vi "DAQ DO.vi"(8 "error in":errorcluster, 10 "on/off":bool, 11 "Alias":string="DO0") -> (0 "error out":errorcluster={"status"=TRUE, "code"=-200099, "source"="DAQmx Create Channel (DO-Digital Output).vi:6970001<append>\n<B>Task Name: </B>_unnamedTask<22>"})   [LabVIEW 2021]
uses:
  Controls/DAQ_Data.ctl
  <vilib>/DAQmx/write.llb/DAQmx Write (Digital Bool 1Line 1Point).vi
  <vilib>/DAQmx/create/channels.llb/DAQmx Create Channel (DO-Digital Output).vi
  <vilib>/DAQmx/miscellaneous.llb/DAQmx Fill In Error Info.vi
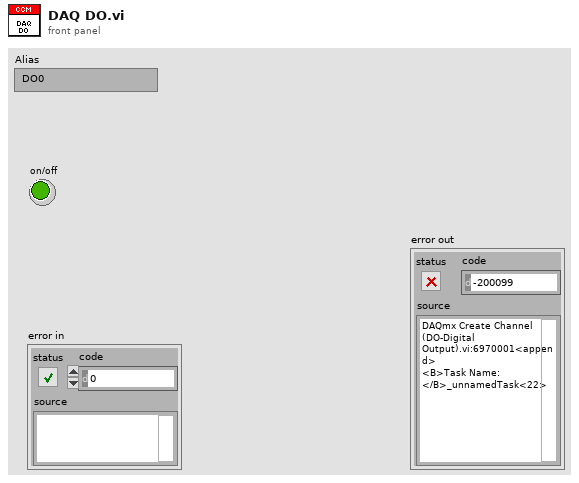
[diagram p1: front panel]
types:
  T1 = typedef "DAQ_Data.ctl" = cluster{"Alias":string, "DAQ Ch":string}
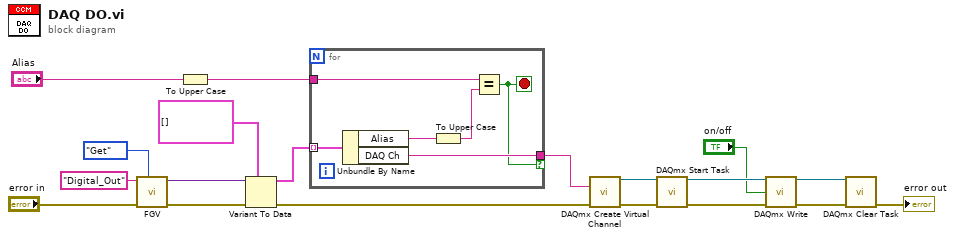
[diagram p0: block diagram]
diagram:
  n1 = call "FGV.vi"("Method (Get)"=enum16{"Get", "Set"}."Get", "error in"="error in", "Name"="Digital_Out") -> ("error out"=w8:errorcluster, "Data out"=w9:variant)  [unwired: 7 in]
  n2 = To Upper Case(1:"Alias") -> (0:w4:string)
  n3 = Variant To Data(error in=w8, type=T1[] [], Variant=w9) -> (data=w5:T1[], error out=w6:errorcluster)
  n4 = for {
    tunnel: w5 -> [w25] mode=indexing
    tunnel: [w24] -> w1 if=w21
    tunnel: w4 -> [w23]
    stop <- w21 stop-if-true
    n5 = Unbundle By Name(w25) -> ("Alias"=w22:string, "DAQ Ch"=w24:string)
    n6 = To Upper Case(1:w22) -> (0:w20:string)
    n7 = Equal?(x=w23, y=w20) -> (x = y?=w21:bool)
  }
  n8 = call-poly <vilib>:"DAQmx Create Virtual Channel.vi"("lines"=w1, "error in"=w6) -> ("task out"=w15:refnum<k21>, "error out"=w16:errorcluster)  [unwired: 12 in]
  n9 = call <vilib>:"DAQmx Start Task.vi"("task/channels in"=w15, "error in"=w16) -> ("task out"=w18:refnum<k21>, "error out"=w17:errorcluster)  [unwired: 12 in]
  n10 = call-poly <vilib>:"DAQmx Write.vi"("task/channels in"=w18, "data"="on/off", "error in"=w17) -> ("task out"=w14:refnum<k21>, "error out"=w13:errorcluster)  [unwired: 10 in, 1 out]
  n11 = call <vilib>:"DAQmx Clear Task.vi"("task in"=w14, "error in"=w13) -> ("error out"=→"error out":errorcluster)  [unwired: 13 in]
